vi "UnregisterMat_Image.vi"(6 "AdressOrData":u64 format="%.0x", 8 "error in":errorcluster, 11 "Image Reference In":T1) -> (0 "error out":errorcluster, 3 "Image Reference Out":T1)   [LabVIEW 2020, in "OpenLvVision_OpenCv.lvlib"]
doc: "Register mat for dll.\nNo malleable to breake vi inlining!"
uses:
  OpenLvVision_OpenCv.lvlib
  <vilib>/OpenLvVision/OpenLvVision_Image/Management/TypeDef/OLV Image.ctl
  <vilib>/OpenLvVision/OpenLvVision_Image/DataAccess/TypeDef/OLV ImagePointer.ctl
  <vilib>/OpenLvVision/OpenLvVision_Image/Management/TypeDef/OLV ImageType.ctl
  <vilib>/OpenLvVision/OpenLvVision_Image/DataAccess/OLV DataAccess.lvlib
  <vilib>/OpenLvVision/OpenLvVision_Image/Management/OLV Management.lvlib
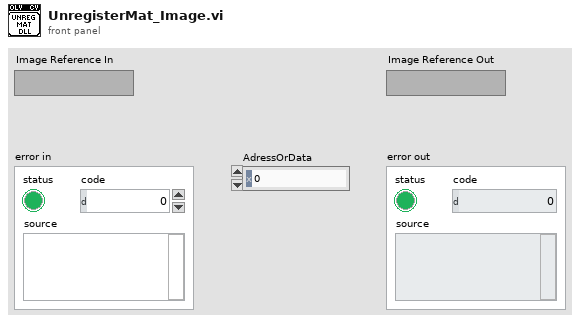
[diagram p1: front panel]
types:
  T1 = typedef "OLV OpenLvVision_Image.lvlib/OLV Management.lvlib/OLV Image.ctl" = refnum<image>
  T2 = typedef "OLV OpenLvVision_Image.lvlib/OLV DataAccess.lvlib/OLV ImagePointer.ctl" = cluster{"ImagePointer":u64, "BorderSize":i32, "LineWidth":i32, "Width":i32, "Height":i32, "ImageFormat":T3}
  T3 = typedef "OLV OpenLvVision_Image.lvlib/OLV Management.lvlib/OLV ImageType.ctl" = enum16{"Mono U8", "Mono U16", "Mono I16", "Mono SGL", "Color U32", "Color U64", "Complex CSG"}
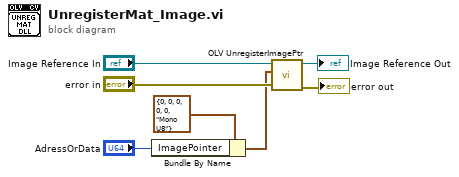
[diagram p0: block diagram]
diagram:
  n1 = Bundle By Name(cluster=T2 {"ImagePointer"=0, "BorderSize"=0, "LineWidth"=0, "Width"=0, "Height"=0, "ImageFormat"=enum."Mono U8"} ("ImagePointer"), "ImagePointer"="AdressOrData") -> (w3:T2)
  n2 = call <vilib>:"OLV UnregisterImagePtr.vi"("error in"="error in", "ImagePointer"=w3, "Image Reference In"="Image Reference In") -> ("error out"=→"error out":errorcluster, "Image Reference Out"=→"Image Reference Out":T1)  [unwired: 7 in]
